vi "Teleop.vi"(10 "Match Info":T1={"Autonomous Elapsed Seconds"=0.0, "TeleOp Elapsed Seconds"=0.0, "Disabled Elapsed Seconds"=0.0, "Visited Autonomous"=FALSE, "Visited TeleOp"=FALSE, "Visited Disabled"=FALSE, "Autonomous Settings"={"Autonomous Style"=enum."Independent", "VI Refnum"=refnum}}, 11 "Call Context":T2) -> ()   [LabVIEW 2014]
doc: "This VI is called for each TeleOp packet received from the DS where the robot is not disabled. It is often used to read from the joysticks and update I/O or to update setpoints for timed control loops. It should complete and return within 20 milliseconds or it may miss DS packets."
uses:
  <vilib>/Rock Robotics/WPI/DriverStation/WPI_DriverStationDerivedRobotMode.ctl
  <vilib>/Rock Robotics/WPI/DriverStation/WPI_DriverStationMatch Info.ctl
  <vilib>/Rock Robotics/WPI/SafetyOutput/WPI_SafetyOutputConfigMenu.ctl
  <vilib>/Rock Robotics/WPI/RobotDrive/WPI_RobotDriveGetSetRefNum.vi
  <vilib>/Rock Robotics/WPI/Joystick/WPI_JoystickGetSetRefNum.vi
  <vilib>/Rock Robotics/Network Tables/SD Read Boolean.vi
  <vilib>/Rock Robotics/Network Tables/SD Read Number.vi
  <vilib>/Rock Robotics/WPI/RobotDrive/WPI_RobotDriveOpen4MotorWithTalon.vi
  <vilib>/Rock Robotics/WPI/RobotDrive/WPI_RobotDriveOpen4MotorWithTalonSRX.vi
  <vilib>/Rock Robotics/WPI/RobotDrive/WPI_RobotDriveOpen4MotorWithCANTalonSRX.vi
  <vilib>/Rock Robotics/WPI/RobotDrive/WPI_RobotDriveOpen4MotorWithVictorSP.vi
  <vilib>/Rock Robotics/WPI/RobotDrive/WPI_RobotDriveOpen4MotorWithVictor.vi
  <vilib>/Rock Robotics/WPI/RobotDrive/WPI_RobotDriveOpen4MotorWithJaguar.vi
  <vilib>/Rock Robotics/WPI/RobotDrive/WPI_RobotDriveOpen4MotorWithCANJaguar.vi
  <vilib>/Rock Robotics/WPI/RobotDrive/WPI_RobotDriveOpen2MotorWithTalon.vi
  <vilib>/Rock Robotics/WPI/RobotDrive/WPI_RobotDriveOpen2MotorWithTalonSRX.vi
  <vilib>/Rock Robotics/WPI/RobotDrive/WPI_RobotDriveOpen2MotorWithCANTalonSRX.vi
  <vilib>/Rock Robotics/WPI/RobotDrive/WPI_RobotDriveOpen2MotorWithVictorSP.vi
  <vilib>/Rock Robotics/WPI/RobotDrive/WPI_RobotDriveOpen2MotorWithVictor.vi
  <vilib>/Rock Robotics/WPI/RobotDrive/WPI_RobotDriveOpen2MotorWithJaguar.vi
  <vilib>/Rock Robotics/WPI/RobotDrive/WPI_RobotDriveOpen2MotorWithCANJaguar.vi
  <vilib>/Rock Robotics/Network Tables/SD Write Numeric Array.vi
  <vilib>/Rock Robotics/Network Tables/SD Write Boolean Array.vi
  <vilib>/Rock Robotics/Network Tables/SD Write Boolean.vi
panel:
  out "Sample Slider 0":dbl(slide) scale=0.0..5.0
  out "Sample Boolean 1":bool
  out "Sample Boolean 0":bool
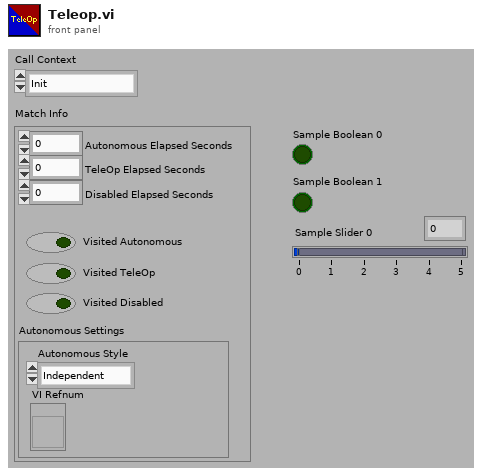
[diagram p1: front panel]
types:
  T1 = typedef "WPI_DriverStationMatch Info.ctl" = cluster{"Autonomous Elapsed Seconds":dbl, "TeleOp Elapsed Seconds":dbl, "Disabled Elapsed Seconds":dbl, "Visited Autonomous":bool, "Visited TeleOp":bool, "Visited Disabled":bool, "Autonomous Settings":cluster{"Autonomous Style":enum16{"Iterative", "Independent"}, "VI Refnum":refnum<vi>}}
  T2 = typedef "WPI_DriverStationDerivedRobotMode.ctl" = enum16{"Init", "Execute", "Stop"}
  T3 = typedef "WPI_JoystickDevRef.ctl" = cluster{"Device":T4}
  T4 = typedef "WPI_JoystickDeviceEnum.ctl" = enum16{"USB 0", "USB 1", "USB 2", "USB 3", "USB 4", "USB 5"}
  T5 = typedef "WPI_RobotDriveDevRef.ctl" = cluster{"DevStatus":errorcluster, "Motors[]":T6[], "Square Inputs":bool, "Max Output":dbl}
  T6 = typedef "WPI_MotorControlDeviceRef.ctl" = cluster{"DeviceStatus":errorcluster, "Type":T7, "PWM":cluster{"Controller":T8, "PWM Channel":T9, "DeadBand":T10}, "CAN":cluster{"Device Number":u8, "Control Mode":T11, "Semaphore":T12, "Max Vout":dbl, "TalonSRX Control Mode":T13}, "Invert":bool, "TransformRef":T14, "InvTransformRef":T14}
  T7 = typedef "WPI_MotorControlType.ctl" = enum16{"PWM", "CAN", "CANTalonSRX"}
  T8 = typedef "FPGA_TypedefDigitalModule.ctl" = enum16{"Controller 1"}
  T9 = typedef "FPGA_DIOPWMChannel.ctl" = enum8{"PWM 0", "PWM 1", "PWM 2", "PWM 3", "PWM 4", "PWM 5", "PWM 6", "PWM 7", "PWM 8", "PWM 9", "PWM MXP 0", "PWM MXP 1", "PWM MXP 2", "PWM MXP 3", "PWM MXP 4", "PWM MXP 5", "PWM MXP 6", "PWM MXP 7", "PWM MXP 8", "PWM MXP 9", "Invalid"}
  T10 = typedef "WPI_PWMDeadband.ctl" = cluster{"Name":string, "maxPositivePwm":i32, "minPositivePwm":i32, "centerPwm":i32, "maxNegativePwm":i32, "minNegativePwm":i32, "angularRange":u16}
  T11 = typedef "WPI_CANJaguar_ControlMode.ctl" = enum8{"Percent VBus", "Current", "Speed", "Position", "Voltage"}
  T12 = typedef "Semaphore RefNum" = refnum<k1>
  T13 = typedef "WPI_CANTalonSRX_APIControlMode.ctl" = enum8{"Percent VBus", "Speed", "Position", "Slave", "Unchanged / Invalid"}
  T14 = typedef "WPI_PWMTransform_ConPane.ctl" = refnum<vi>
  T15 = typedef "WPI_SafetyOutputConfigMenu.ctl" = enum16{"Enable", "Disable"}
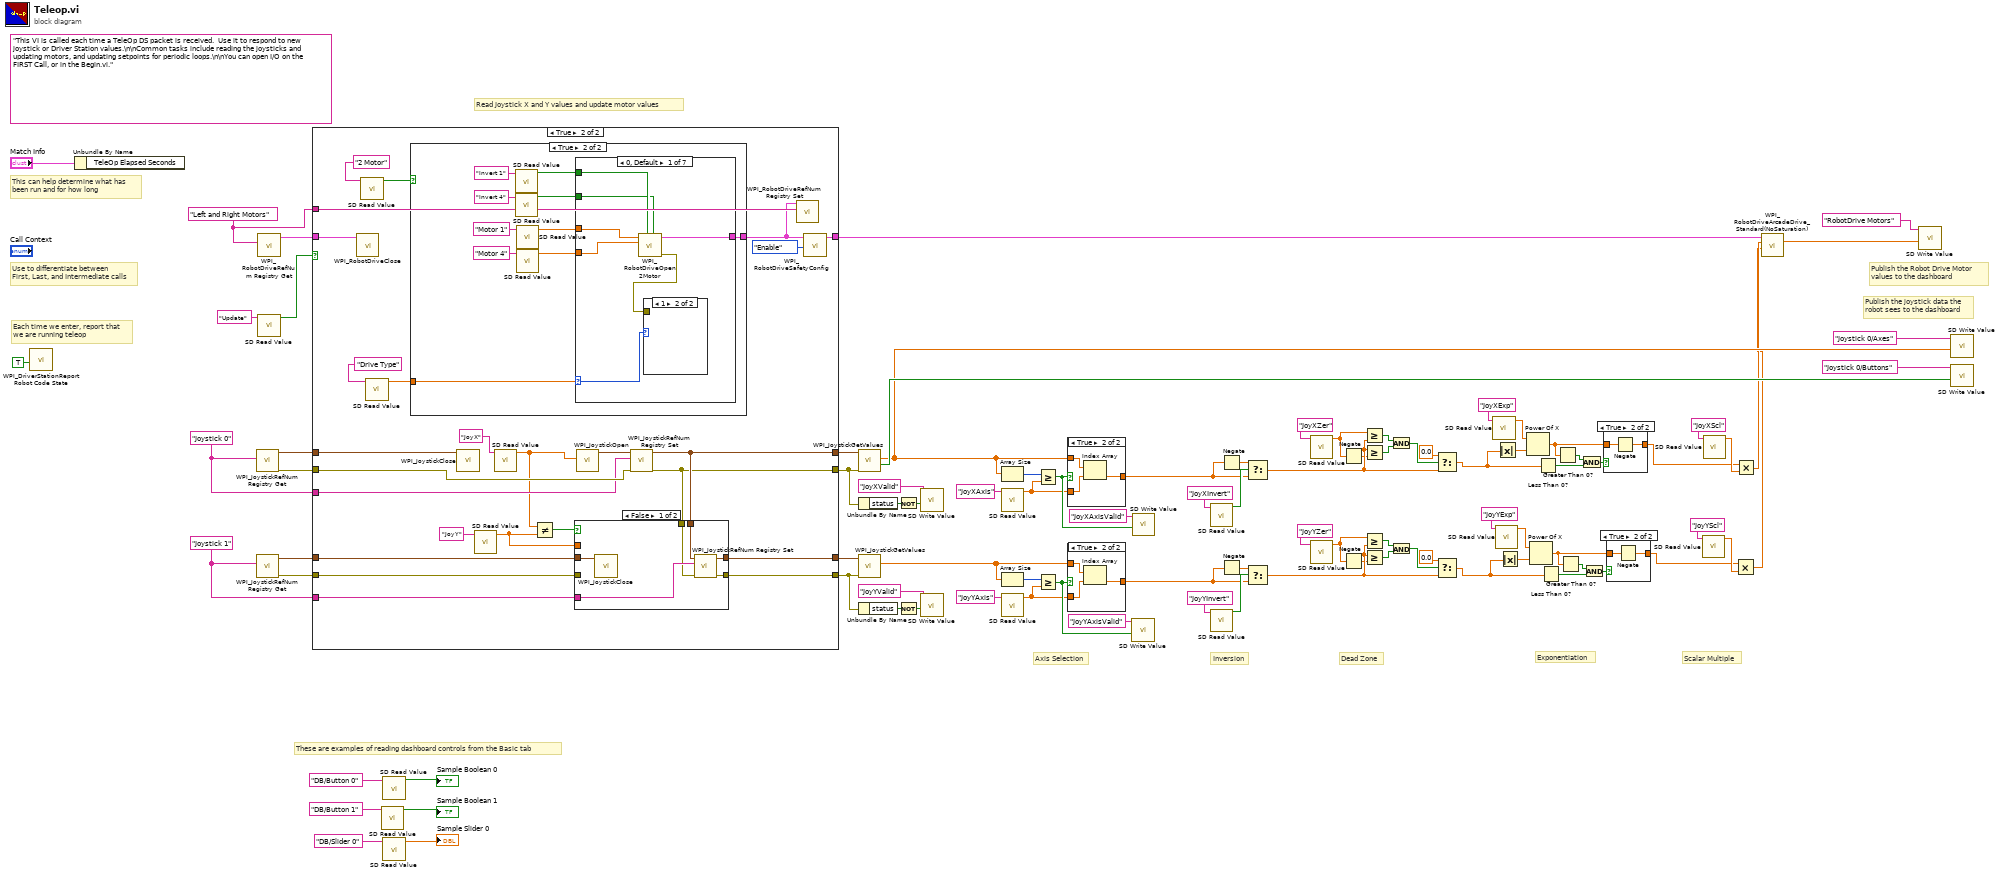
[diagram p0: block diagram]
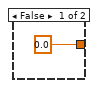
[diagram p4: hidden frame]
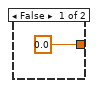
[diagram p5: hidden frame]
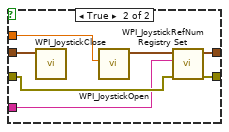
[diagram p7: hidden frame]
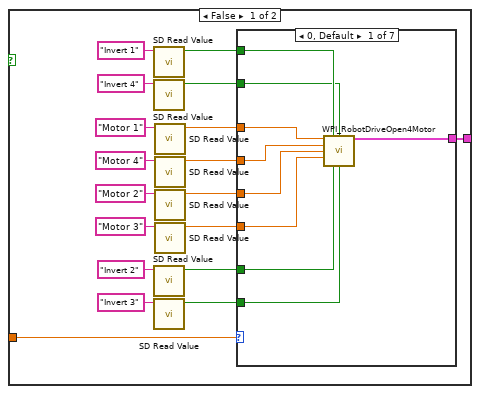
[diagram p8: hidden frame]
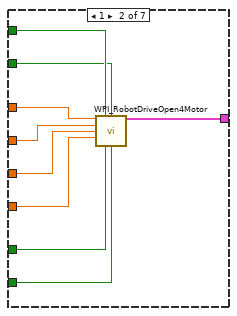
[diagram p9: hidden frame]
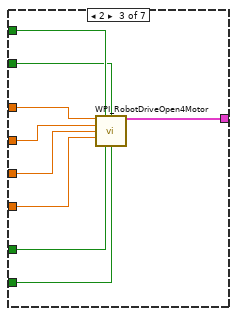
[diagram p10: hidden frame]
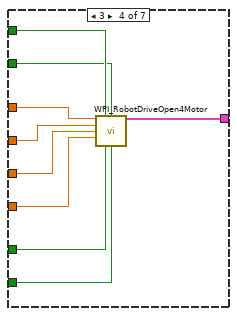
[diagram p11: hidden frame]
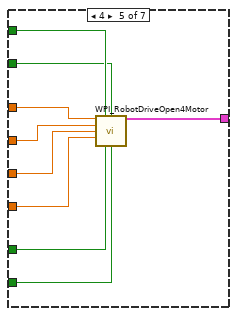
[diagram p12: hidden frame]
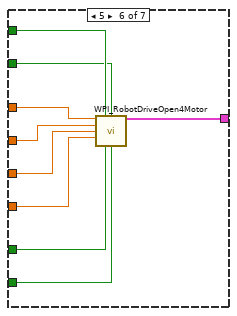
[diagram p13: hidden frame]
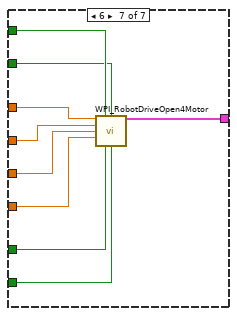
[diagram p14: hidden frame]
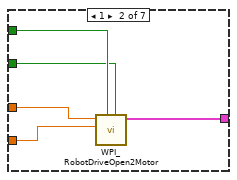
[diagram p16: hidden frame]
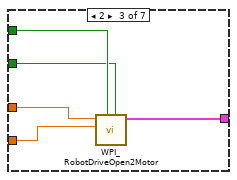
[diagram p17: hidden frame]
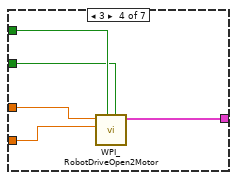
[diagram p18: hidden frame]
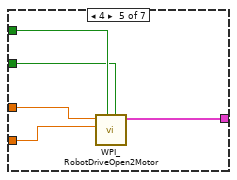
[diagram p19: hidden frame]
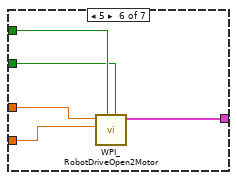
[diagram p20: hidden frame]
diagram:
  w73 = "Joystick 1" ("refnum name")
  (unwired) "This VI is called each time a TeleOp DS packet is received.  Use it to respond to new joystick or Driver Station values.\n\nCommon tasks include reading the joysticks and updating motors, and updating setpoints for periodic loops.\n\nYou can open I/O on the FIRST Call, or in the Begin.vi."
  w75 = "Joystick 0" ("refnum name")
  w76 = "Left and Right Motors" ("refnum name")
  # "Exponentiation"
  # "Scalar Multiple"
  # "Dead Zone"
  # "Inversion"
  # "Axis Selection"
  # "These are examples of reading dashboard controls from the Basic tab"
  # "Publish the Robot Drive Motor\nvalues to the dashboard"
  # "Publish the joystick data the\nrobot sees to the dashboard"
  # "Each time we enter, report that\nwe are running teleop"
  # "Use to differentiate between\nFirst, Last, and Intermediate calls"
  # "This can help determine what has\nbeen run and for how long"
  # "Read Joystick X and Y values and update motor values"
  n1 = call <vilib>:"WPI_DriverStationReport Robot Code State.vi"("TeleOp"=TRUE ("Autonomous")) -> ()  [unwired: 10 in, 1 out]
  n2 = Unbundle By Name("Match Info") -> ()  [unwired: 1 out]
  n3 = call <vilib>:"WPI_JoystickRefNum Registry Get.vi"("refnum name"=w75) -> ("error out"=w74:errorcluster, "JoystickDevRef"=w79:T3)  [unwired: 1 in, 8 out]
  n4 = call <vilib>:"WPI_JoystickRefNum Registry Get.vi"("refnum name"=w73) -> ("error out"=w71:errorcluster, "JoystickDevRef"=w72:T3)  [unwired: 1 in, 8 out]
  n5 = call <vilib>:"WPI_RobotDriveRefNum Registry Get.vi"("refnum name"=w76) -> ("RobotDriveDevRef"=w81:T5)  [unwired: 1 in, 9 out]
  n6 = call-poly <vilib>:"SD Read Value.vi"("Name"="Update") -> ("Boolean"=w78:bool)  [unwired: 8 in, 2 out]
  n7 = case shown="True" w78 {
    tunnel: w81 -> [w99 w115]
    tunnel: [w99 w120] -> w80
    tunnel: w79 -> [w98 w114]
    tunnel: w76 -> [_ w117]
    tunnel: w75 -> [_ w112]
    tunnel: w74 -> [w97 w121]
    tunnel: w73 -> [_ w108]
    tunnel: w72 -> [w96 w110]
    tunnel: w71 -> [w95 w109]
    tunnel: [w98 w103] -> w70
    tunnel: [w97 w102] -> w67
    tunnel: [w96 w101] -> w69
    tunnel: [w95 w100] -> w64
    frame False {
    }
    frame True {
      n8 = call <vilib>:"WPI_RobotDriveClose.vi"("RobotDriveDevRef"=w115) -> ()  [unwired: 10 in, 1 out]
      n9 = call-poly <vilib>:"SD Read Value.vi"("Name"="2 Motor") -> ("Boolean"=w123:bool)  [unwired: 8 in, 2 out]
      n10 = call-poly <vilib>:"SD Read Value.vi"("Name"="Drive Type") -> ("Numeric"=w118:dbl)  [unwired: 8 in, 2 out]
      n11 = case shown="True" w123 {
        tunnel: [w155 w228] -> w116
        tunnel: w118 -> [w154 w227]
        frame False {
          n12 = call-poly <vilib>:"SD Read Value.vi"("Name"="Invert 1") -> ("Boolean"=w146:bool)  [unwired: 8 in, 2 out]
          n13 = call-poly <vilib>:"SD Read Value.vi"("Name"="Invert 4") -> ("Boolean"=w145:bool)  [unwired: 8 in, 2 out]
          n14 = call-poly <vilib>:"SD Read Value.vi"("Name"="Invert 2") -> ("Boolean"=w144:bool)  [unwired: 8 in, 2 out]
          n15 = call-poly <vilib>:"SD Read Value.vi"("Name"="Invert 3") -> ("Boolean"=w143:bool)  [unwired: 8 in, 2 out]
          n16 = call-poly <vilib>:"SD Read Value.vi"("Name"="Motor 1") -> ("Numeric"=w142:dbl)  [unwired: 8 in, 2 out]
          n17 = call-poly <vilib>:"SD Read Value.vi"("Name"="Motor 4") -> ("Numeric"=w141:dbl)  [unwired: 8 in, 2 out]
          n18 = call-poly <vilib>:"SD Read Value.vi"("Name"="Motor 2") -> ("Numeric"=w140:dbl)  [unwired: 8 in, 2 out]
          n19 = call-poly <vilib>:"SD Read Value.vi"("Name"="Motor 3") -> ("Numeric"=w139:dbl)  [unwired: 8 in, 2 out]
          n20 = case shown="0, Default" w154 {
            tunnel: [w164 w173 w182 w191 w200 w209 w218] -> w155
            tunnel: w146 -> [w163 w172 w181 w190 w199 w208 w217]
            tunnel: w145 -> [w162 w171 w180 w189 w198 w207 w216]
            tunnel: w144 -> [w161 w170 w179 w188 w197 w206 w215]
            tunnel: w143 -> [w160 w169 w178 w187 w196 w205 w214]
            tunnel: w142 -> [w159 w168 w177 w186 w195 w204 w213]
            tunnel: w141 -> [w158 w167 w176 w185 w194 w203 w212]
            tunnel: w140 -> [w157 w166 w175 w184 w193 w202 w211]
            tunnel: w139 -> [w156 w165 w174 w183 w192 w201 w210]
            frame 0, Default {
              n21 = call-poly <vilib>:"WPI_RobotDriveOpen4Motor.vi"("Rear Left Motor"=w159, "Rear Left Motor Inverted"=w163, "Rear Right Motor Inverted"=w162, "Rear Right Motor"=w158, "Front Left Motor"=w157, "Front Right Motor"=w156, "Front Left Motor Inverted"=w161, "Front Right Motor Inverted"=w160) -> ("RobotDriveDevRef"=w164:T5)  [unwired: 6 in, 1 out]
            }
            frame 1 {
              n22 = call-poly <vilib>:"WPI_RobotDriveOpen4Motor.vi"("Rear Left Motor"=w168, "Rear Left Motor Inverted"=w172, "Rear Right Motor Inverted"=w171, "Rear Right Motor"=w167, "Front Left Motor"=w166, "Front Right Motor"=w165, "Front Left Motor Inverted"=w170, "Front Right Motor Inverted"=w169) -> ("RobotDriveDevRef"=w173:T5)  [unwired: 6 in, 1 out]
            }
            frame 2 {
              n23 = call-poly <vilib>:"WPI_RobotDriveOpen4Motor.vi"("Rear Left Motor"=w177, "Rear Left Motor Inverted"=w181, "Rear Right Motor Inverted"=w180, "Rear Right Motor"=w176, "Front Left Motor"=w175, "Front Right Motor"=w174, "Front Left Motor Inverted"=w179, "Front Right Motor Inverted"=w178) -> ("RobotDriveDevRef"=w182:T5)  [unwired: 6 in, 1 out]
            }
            frame 3 {
              n24 = call-poly <vilib>:"WPI_RobotDriveOpen4Motor.vi"("Rear Left Motor"=w186, "Rear Left Motor Inverted"=w190, "Rear Right Motor Inverted"=w189, "Rear Right Motor"=w185, "Front Left Motor"=w184, "Front Right Motor"=w183, "Front Left Motor Inverted"=w188, "Front Right Motor Inverted"=w187) -> ("RobotDriveDevRef"=w191:T5)  [unwired: 6 in, 1 out]
            }
            frame 4 {
              n25 = call-poly <vilib>:"WPI_RobotDriveOpen4Motor.vi"("Rear Left Motor"=w195, "Rear Left Motor Inverted"=w199, "Rear Right Motor Inverted"=w198, "Rear Right Motor"=w194, "Front Left Motor"=w193, "Front Right Motor"=w192, "Front Left Motor Inverted"=w197, "Front Right Motor Inverted"=w196) -> ("RobotDriveDevRef"=w200:T5)  [unwired: 6 in, 1 out]
            }
            frame 5 {
              n26 = call-poly <vilib>:"WPI_RobotDriveOpen4Motor.vi"("Rear Left Motor"=w204, "Rear Left Motor Inverted"=w208, "Rear Right Motor Inverted"=w207, "Rear Right Motor"=w203, "Front Left Motor"=w202, "Front Right Motor"=w201, "Front Left Motor Inverted"=w206, "Front Right Motor Inverted"=w205) -> ("RobotDriveDevRef"=w209:T5)  [unwired: 6 in, 1 out]
            }
            frame 6 {
              n27 = call-poly <vilib>:"WPI_RobotDriveOpen4Motor.vi"("Rear Left Motor"=w213, "Rear Left Motor Inverted"=w217, "Rear Right Motor Inverted"=w216, "Rear Right Motor"=w212, "Front Left Motor"=w211, "Front Right Motor"=w210, "Front Left Motor Inverted"=w215, "Front Right Motor Inverted"=w214) -> ("RobotDriveDevRef"=w218:T5)  [unwired: 6 in, 1 out]
            }
          }
        }
        frame True {
          n28 = call-poly <vilib>:"SD Read Value.vi"("Name"="Invert 1") -> ("Boolean"=w222:bool)  [unwired: 8 in, 2 out]
          n29 = call-poly <vilib>:"SD Read Value.vi"("Name"="Invert 4") -> ("Boolean"=w221:bool)  [unwired: 8 in, 2 out]
          n30 = call-poly <vilib>:"SD Read Value.vi"("Name"="Motor 1") -> ("Numeric"=w220:dbl)  [unwired: 8 in, 2 out]
          n31 = call-poly <vilib>:"SD Read Value.vi"("Name"="Motor 4") -> ("Numeric"=w219:dbl)  [unwired: 8 in, 2 out]
          n32 = case shown="0, Default" w227 {
            selector: w227 -> [w229 _ _ _ _ _ _]
            tunnel: [w235 w240 w245 w250 w255 w260 w265] -> w228
            tunnel: w222 -> [w234 w239 w244 w249 w254 w259 w264]
            tunnel: w221 -> [w233 w238 w243 w248 w253 w258 w263]
            tunnel: w220 -> [w232 w237 w242 w247 w252 w257 w262]
            tunnel: w219 -> [w231 w236 w241 w246 w251 w256 w261]
            frame 0, Default {
              n33 = call-poly <vilib>:"WPI_RobotDriveOpen2Motor.vi"("Right Motor Inverted"=w233, "Left Motor Inverted"=w234, "Right Motor"=w231, "Left Motor"=w232) -> ("error out"=w230:errorcluster, "RobotDriveDevRef"=w235:T5)  [unwired: 6 in]
              n34 = case shown="1" w229 {
                tunnel: w230 -> [_ _]
                frame 0, Default {
                }
                frame 1 {
                }
              }
            }
            frame 1 {
              n35 = call-poly <vilib>:"WPI_RobotDriveOpen2Motor.vi"("Right Motor Inverted"=w238, "Left Motor Inverted"=w239, "Right Motor"=w236, "Left Motor"=w237) -> ("RobotDriveDevRef"=w240:T5)  [unwired: 6 in, 1 out]
            }
            frame 2 {
              n36 = call-poly <vilib>:"WPI_RobotDriveOpen2Motor.vi"("Right Motor Inverted"=w243, "Left Motor Inverted"=w244, "Right Motor"=w241, "Left Motor"=w242) -> ("RobotDriveDevRef"=w245:T5)  [unwired: 6 in, 1 out]
            }
            frame 3 {
              n37 = call-poly <vilib>:"WPI_RobotDriveOpen2Motor.vi"("Right Motor Inverted"=w248, "Left Motor Inverted"=w249, "Right Motor"=w246, "Left Motor"=w247) -> ("RobotDriveDevRef"=w250:T5)  [unwired: 6 in, 1 out]
            }
            frame 4 {
              n38 = call-poly <vilib>:"WPI_RobotDriveOpen2Motor.vi"("Right Motor Inverted"=w253, "Left Motor Inverted"=w254, "Right Motor"=w251, "Left Motor"=w252) -> ("RobotDriveDevRef"=w255:T5)  [unwired: 6 in, 1 out]
            }
            frame 5 {
              n39 = call-poly <vilib>:"WPI_RobotDriveOpen2Motor.vi"("Right Motor Inverted"=w258, "Left Motor Inverted"=w259, "Right Motor"=w256, "Left Motor"=w257) -> ("RobotDriveDevRef"=w260:T5)  [unwired: 6 in, 1 out]
            }
            frame 6 {
              n40 = call-poly <vilib>:"WPI_RobotDriveOpen2Motor.vi"("Right Motor Inverted"=w263, "Left Motor Inverted"=w264, "Right Motor"=w261, "Left Motor"=w262) -> ("RobotDriveDevRef"=w265:T5)  [unwired: 6 in, 1 out]
            }
          }
        }
      }
      n41 = call <vilib>:"WPI_JoystickClose.vi"("JoystickDevRef"=w114) -> ()  [unwired: 11 in]
      n42 = call-poly <vilib>:"SD Read Value.vi"("Name"="JoyY") -> ("Numeric"=w104:dbl)  [unwired: 8 in, 2 out]
      n43 = call-poly <vilib>:"SD Read Value.vi"("Name"="JoyX") -> ("Numeric"=w106:dbl)  [unwired: 8 in, 2 out]
      n44 = Not Equal?(x=w106, y=w104) -> (x != y?=w105:bool)
      n45 = call <vilib>:"WPI_JoystickOpen.vi"("JoystickDevice"=w106) -> ("JoystickDevRef"=w113:T3)  [unwired: 10 in]
      n46 = call <vilib>:"WPI_JoystickRefNum Registry Set.vi"("error in (no error)"=w121, "refnum name"=w112, "JoystickDevRef"=w113) -> ("error out"=w102:errorcluster, "JoystickDevRef"=w103:T3)  [unwired: 7 in]
      n47 = case shown="False" w105 {
        tunnel: w110 -> [w129 w136]
        tunnel: w109 -> [_ w135]
        tunnel: w108 -> [w130 w134]
        tunnel: w104 -> [_ w133]
        tunnel: w103 -> [w126 _]
        tunnel: w102 -> [w125 _]
        tunnel: [w128 w132] -> w101
        tunnel: [w127 w131] -> w100
        frame False {
          n48 = call <vilib>:"WPI_JoystickClose.vi"("JoystickDevRef"=w129) -> ()  [unwired: 11 in]
          n49 = call <vilib>:"WPI_JoystickRefNum Registry Set.vi"("error in (no error)"=w125, "refnum name"=w130, "JoystickDevRef"=w126) -> ("error out"=w127:errorcluster, "JoystickDevRef"=w128:T3)  [unwired: 7 in]
        }
        frame True {
          n50 = call <vilib>:"WPI_JoystickClose.vi"("JoystickDevRef"=w136) -> ()  [unwired: 11 in]
          n51 = call <vilib>:"WPI_JoystickOpen.vi"("JoystickDevice"=w133) -> ("JoystickDevRef"=w137:T3)  [unwired: 10 in]
          n52 = call <vilib>:"WPI_JoystickRefNum Registry Set.vi"("error in (no error)"=w135, "refnum name"=w134, "JoystickDevRef"=w137) -> ("error out"=w131:errorcluster, "JoystickDevRef"=w132:T3)  [unwired: 7 in]
        }
      }
      n53 = call <vilib>:"WPI_RobotDriveRefNum Registry Set.vi"("refnum name"=w117, "RobotDriveDevRef"=w116) -> ()  [unwired: 8 in, 2 out]
      n54 = call <vilib>:"WPI_RobotDriveSafetyConfig.vi"("mode"=WPI_SafetyOutputConfigMenu."Enable", "RobotDriveDevRef"=w116) -> ("RobotDriveDevRef"=w120:T5)  [unwired: 8 in, 1 out]
    }
  }
  n55 = call-poly <vilib>:"SD Read Value.vi"("Name"="DB/Button 1" ("refnum name")) -> ("Boolean"=→"Sample Boolean 1":bool)  [unwired: 8 in, 2 out]
  n56 = call-poly <vilib>:"SD Read Value.vi"("Name"="DB/Button 0" ("refnum name")) -> ("Boolean"=→"Sample Boolean 0":bool)  [unwired: 8 in, 2 out]
  n57 = call-poly <vilib>:"SD Read Value.vi"("Name"="DB/Slider 0" ("refnum name")) -> ("Numeric"=→"Sample Slider 0":dbl)  [unwired: 8 in, 2 out]
  n58 = call <vilib>:"WPI_JoystickGetValues.vi"("error in (no error)"=w67, "JoystickDevRef"=w70) -> ("Buttons"=w82:bool[], "Axes"=w62:dbl[])  [unwired: 5 in, 3 out]
  n59 = Unbundle By Name(w67) -> ("status"=w31:bool)
  n60 = call <vilib>:"WPI_JoystickGetValues.vi"("error in (no error)"=w64, "JoystickDevRef"=w69) -> ("Axes"=w53:dbl[])  [unwired: 5 in, 4 out]
  n61 = Unbundle By Name(w64) -> ("status"=w33:bool)
  n62 = Not(x=w31) -> (.not. x?=w32:bool)
  n63 = Not(x=w33) -> (.not. x?=w34:bool)
  n64 = call-poly <vilib>:"SD Write Value.vi"("Boolean"=w32, "Name"="JoyXValid") -> ()  [unwired: 8 in, 2 out]
  n65 = call-poly <vilib>:"SD Write Value.vi"("Boolean"=w34, "Name"="JoyYValid") -> ()  [unwired: 8 in, 2 out]
  n66 = Array Size(array=w62) -> (size(s)=w63:i32)
  n67 = call-poly <vilib>:"SD Read Value.vi"("Name"="JoyXAxis") -> ("Numeric"=w59:dbl)  [unwired: 8 in, 2 out]
  n68 = Array Size(array=w53) -> (size(s)=w57:i32)
  n69 = call-poly <vilib>:"SD Read Value.vi"("Name"="JoyYAxis") -> ("Numeric"=w54:dbl)  [unwired: 8 in, 2 out]
  n70 = Greater Or Equal?(x=w63, y=w59) -> (x >= y?=w60:bool)
  n71 = Greater Or Equal?(x=w57, y=w54) -> (x >= y?=w55:bool)
  n72 = case shown="True" w60 {
    tunnel: w62 -> [_ w269]
    tunnel: w59 -> [_ w268]
    tunnel: [0.0 ("upper limit") w267] -> w47
    frame False {
    }
    frame True {
      n73 = Index Array(array=w269, index=w268) -> (element=w267:dbl)
    }
  }
  n74 = case shown="True" w55 {
    tunnel: w53 -> [_ w273]
    tunnel: w54 -> [_ w272]
    tunnel: [0.0 ("upper limit") w271] -> w35
    frame False {
    }
    frame True {
      n75 = Index Array(array=w273, index=w272) -> (element=w271:dbl)
    }
  }
  n76 = call-poly <vilib>:"SD Write Value.vi"("Boolean"=w55, "Name"="JoyYAxisValid") -> ()  [unwired: 8 in, 2 out]
  n77 = call-poly <vilib>:"SD Write Value.vi"("Boolean"=w60, "Name"="JoyXAxisValid") -> ()  [unwired: 8 in, 2 out]
  n78 = call-poly <vilib>:"SD Read Value.vi"("Name"="JoyXInvert") -> ("Boolean"=w49:bool)  [unwired: 8 in, 2 out]
  n79 = call-poly <vilib>:"SD Read Value.vi"("Name"="JoyYInvert") -> ("Boolean"=w40:bool)  [unwired: 8 in, 2 out]
  n80 = Negate(x=w47) -> (-x=w48:dbl)
  n81 = Negate(x=w35) -> (-x=w39:dbl)
  n82 = Select(t=w48, s=w49, f=w47) -> (s? t:f=w46:dbl)
  n83 = Select(t=w39, s=w40, f=w35) -> (s? t:f=w38:dbl)
  n84 = call-poly <vilib>:"SD Read Value.vi"("Name"="JoyXZer") -> ("Numeric"=w26:dbl)  [unwired: 8 in, 2 out]
  n85 = call-poly <vilib>:"SD Read Value.vi"("Name"="JoyYZer") -> ("Numeric"=w19:dbl)  [unwired: 8 in, 2 out]
  n86 = Negate(x=w26) -> (-x=w27:dbl)
  n87 = Negate(x=w19) -> (-x=w20:dbl)
  n88 = Greater Or Equal?(x=w26, y=w46) -> (x >= y?=w29:bool)
  n89 = Greater Or Equal?(x=w46, y=w27) -> (x >= y?=w28:bool)
  n90 = Greater Or Equal?(x=w19, y=w38) -> (x >= y?=w22:bool)
  n91 = Greater Or Equal?(x=w38, y=w20) -> (x >= y?=w21:bool)
  n92 = And(x=w29, y=w28) -> (x .and. y?=w25:bool)
  n93 = And(x=w22, y=w21) -> (x .and. y?=w18:bool)
  n94 = Select(t=0.0, s=w25, f=w46) -> (s? t:f=w6:dbl)
  n95 = Select(t=0.0, s=w18, f=w38) -> (s? t:f=w1:dbl)
  n96 = call-poly <vilib>:"SD Read Value.vi"("Name"="JoyXExp") -> ("Numeric"=w44:dbl)  [unwired: 8 in, 2 out]
  n97 = call-poly <vilib>:"SD Read Value.vi"("Name"="JoyYExp") -> ("Numeric"=w36:dbl)  [unwired: 8 in, 2 out]
  n98 = Absolute Value(x=w6) -> (abs(x)=w8:dbl)
  n99 = Absolute Value(x=w1) -> (abs(x)=w7:dbl)
  n100 = Power Of X(1:w8, 2:w44) -> (0:w13:dbl)
  n101 = Power Of X(1:w7, 2:w36) -> (0:w9:dbl)
  n102 = Less Than 0?(x=w6) -> (x < 0?=w15:bool)
  n103 = Less Than 0?(x=w1) -> (x < 0?=w11:bool)
  n104 = Greater Than 0?(x=w13) -> (x > 0?=w14:bool)
  n105 = Greater Than 0?(x=w9) -> (x > 0?=w10:bool)
  n106 = And(x=w14, y=w15) -> (x .and. y?=w16:bool)
  n107 = And(x=w10, y=w11) -> (x .and. y?=w12:bool)
  n108 = case shown="True" w16 {
    tunnel: w13 -> [w274 w275]
    tunnel: [w274 w276] -> w5
    frame False {
    }
    frame True {
      n109 = Negate(x=w275) -> (-x=w276:dbl)
    }
  }
  n110 = case shown="True" w12 {
    tunnel: w9 -> [w277 w278]
    tunnel: [w277 w279] -> w3
    frame False {
    }
    frame True {
      n111 = Negate(x=w278) -> (-x=w279:dbl)
    }
  }
  n112 = call-poly <vilib>:"SD Read Value.vi"("Name"="JoyYScl") -> ("Numeric"=w37:dbl)  [unwired: 8 in, 2 out]
  n113 = call-poly <vilib>:"SD Read Value.vi"("Name"="JoyXScl") -> ("Numeric"=w45:dbl)  [unwired: 8 in, 2 out]
  n114 = Multiply(x=w3, y=w37) -> (x*y=w2:dbl)
  n115 = Multiply(x=w5, y=w45) -> (x*y=w4:dbl)
  n116 = call <vilib>:"WPI_RobotDriveArcadeDrive_Standard(NoSaturation).vi"("Y axis value"=w2, "X axis value"=w4, "RobotDriveDevRef"=w80) -> ("Motor Values"=w85:dbl[])  [unwired: 1 in, 7 out]
  n117 = call-poly <vilib>:"SD Write Value.vi"("Numeric Array"=w85, "Name"="RobotDrive Motors") -> ()  [unwired: 8 in, 2 out]
  n118 = call-poly <vilib>:"SD Write Value.vi"("Numeric Array"=w62, "Name"="Joystick 0/Axes") -> ()  [unwired: 8 in, 2 out]
  n119 = call-poly <vilib>:"SD Write Value.vi"("Boolean Array"=w82, "Name"="Joystick 0/Buttons") -> ()  [unwired: 8 in, 2 out]
